vi "RecrystalliseSendAHKLow.vi"() -> ()   [LabVIEW 2017]
panel:
  out "timed out?":bool
  out "error out":errorcluster
  in  "error in (no error)":errorcluster
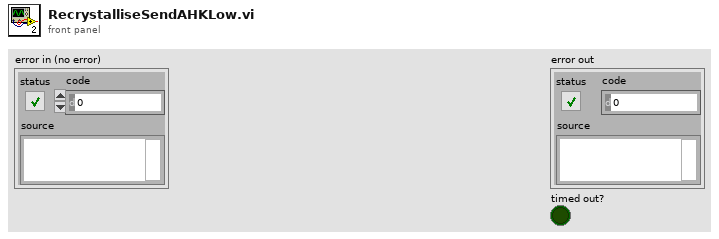
[diagram p1: front panel]
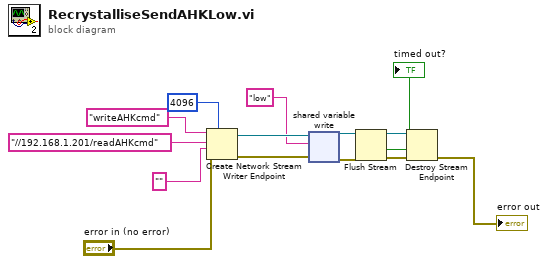
[diagram p0: block diagram]
diagram:
  n1 = Create Network Stream Writer Endpoint(7:4096 ("writer buffer size"), 8:"error in (no error)", 9:"", 10:"//192.168.1.201/readAHKcmd" ("reader url"), 11:"writeAHKcmd" ("writer name")) -> (0:w9:errorcluster, 3:w10:refnum<k21>)  [unwired: 2 in]
  n2 = shared-variable-write(w10, w9, "low" ("data in")) -> (w3:refnum<k21>, w6:errorcluster)  [unwired: 1 in, 1 out]
  n3 = Flush Stream(8:w6, 11:w3) -> (0:w5:errorcluster, 1:→"timed out?":bool, 3:w4:refnum<k21>)  [unwired: 2 in]
  n4 = Destroy Stream Endpoint(8:w5, 11:w4) -> (0:→"error out":errorcluster)
